vi "update channels to type def.vi"(11 "fixed channel configuration in":refnum<class "control module configuration.lvclass">) -> (3 "fixed channel configuration out":refnum<class "control module configuration.lvclass">)   [LabVIEW 2013, in "control module configuration.lvclass"]
uses:
  control module configuration.lvclass
  control module configuration.lvclass/control module configuration.ctl
  <vilib>/NI/Tag Bus/tag/tag descriptor.lvclass/tag descriptor.ctl
  <vilib>/NI/Tag Bus Module Framework/channel/TBM channel.lvclass/TBM channel.ctl
  <vilib>/NI/Tag Bus/tag/read data type.vi
  <vilib>/NI/Tag Bus Module Framework/channel/Read channel classification.vi
  <vilib>/NI/Tag Bus/tag/read tag name.vi
  <vilib>/NI/Tag Bus/tag/tag descriptor.lvclass
  <vilib>/NI/Tag Bus Module Framework/channel/TBM channel.lvclass
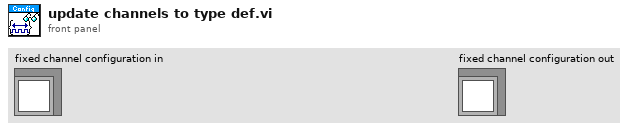
[diagram p1: front panel]
types:
  T1 = typedef "tag bus.lvlib/tag descriptor.lvclass/Data Type.ctl" = enum16{"Double", "Single", "I64", "I32", "I16", "I8", "U64", "U32", "U16", "U8", "Boolean", "String", "Array of Double", "Array of Single", "Array of I64", "Array of I32", "Array of I16", "Array of I8", "Array of U64", "Array of U32", "Array of U16", "Array of U8", "Array of Boolean", "Array of String"}
  T2 = typedef "TBM channel.lvclass/channel classification.ctl" = enum16{"input data", "output data", "processing parameter", "processing result"}
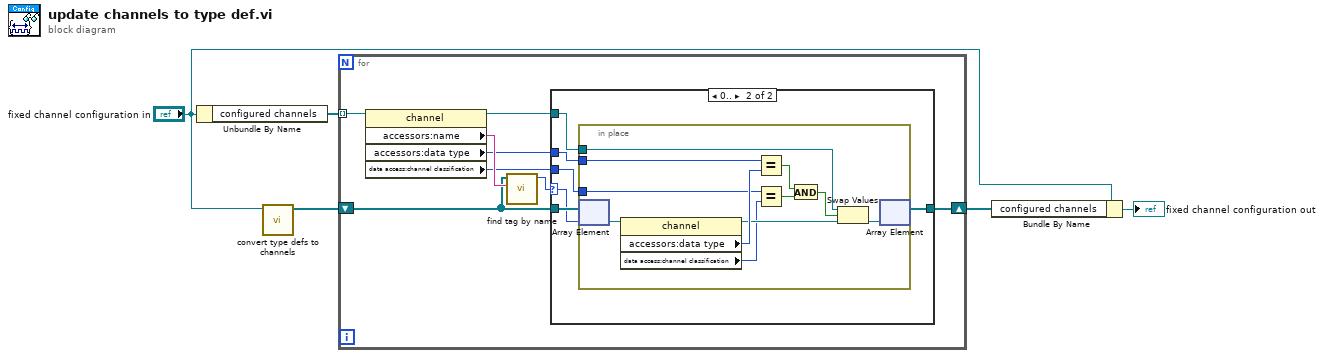
[diagram p0: block diagram]
diagram:
  n1 = Unbundle By Name("fixed channel configuration in") -> ("configured channels"=w2:refnum<class "TBM channel.lvclass">[])
  n2 = call "convert type defs to channels.vi"("fixed channel configuration"="fixed channel configuration in") -> ("Array out"=w4:refnum<class "TBM channel.lvclass">[])  [unwired: 9 in, 1 out]
  n3 = for {
    shift-right: [w9] -> w3
    shift-left: w4 -> [w10]
    tunnel: w2 -> [w13] mode=indexing
    n4 = property class="channel"(reference=w13) -> (reference out=w7:refnum<class "TBM channel.lvclass">, "accessors:name"=w12:string, "accessors:data type"=w8:T1, "data access:channel classification"=w6:T2)  [unwired: 1 in, 1 out]
    n5 = call <vilib>:"find tag by name.vi"("name"=w12, "tags in"=w10) -> ("index"=w11:i32)  [unwired: 9 in]
    n6 = case shown="0.." w11 {
      selector: w11 -> [_ w19]
      tunnel: w10 -> [w14 w20]
      tunnel: [w14 w18] -> w9
      tunnel: w8 -> [_ w17]
      tunnel: w7 -> [_ w16]
      tunnel: w6 -> [_ w15]
      frame ..-1 {
      }
      frame 0.. {
        n7 = in-place {
          in-place-border: w17 -> [w29]
          in-place-border: w16 -> [w26]
          in-place-border: w15 -> [w24]
          n8 = in-place-array #1(w20, w19) -> (w31:refnum<class "TBM channel.lvclass">)
          n9 = property class="channel"(reference=w31) -> (reference out=w28:refnum<class "TBM channel.lvclass">, "accessors:data type"=w30:T1, "data access:channel classification"=w21:T2)  [unwired: 1 in, 1 out]
          n10 = Equal?(x=w29, y=w30) -> (x = y?=w25:bool)
          n11 = Equal?(x=w24, y=w21) -> (x = y?=w22:bool)
          n12 = And(x=w25, y=w22) -> (x .and. y?=w23:bool)
          n13 = Swap Values(12:w26, 13:w23, 14:w28) -> (3:w27:refnum<class "TBM channel.lvclass">)  [unwired: 1 out]
          n14 = in-place-array #1(w27) -> (w18:refnum<class "TBM channel.lvclass">[])  [unwired: 1 out]
        }
      }
    }
  }
  n15 = Bundle By Name(cluster="fixed channel configuration in", "configured channels"=w3) -> (→"fixed channel configuration out":refnum<class "control module configuration.lvclass">)
